vi "Timer Get Time.vi"(8 "error in (no error)":errorcluster, 11 "Timer reference":refnum<data-value>) -> (0 "error out":errorcluster, 1 "Running ?":bool, 2 "Elapsed Time (ms)":u32, 3 "Timer reference  out":refnum<data-value>)   [LabVIEW 2018]
doc: "This VI is part of a Timer class that is implemented with the DVR. It returns current values of the timer while the Timer is running.\n\nAAL 9/09"
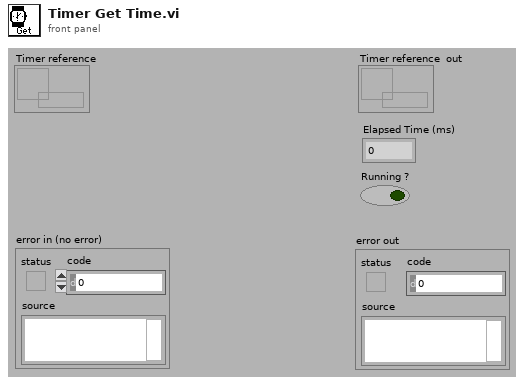
[diagram p1: front panel]
types:
  T1 = cluster{"Start Time":i32, "Elapsed Time":i32, "Running?":bool}
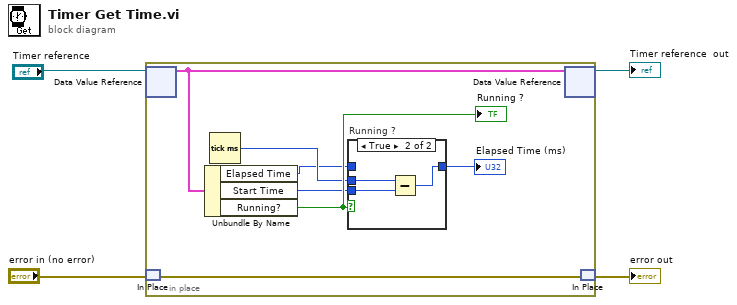
[diagram p0: block diagram]
diagram:
  n1 = in-place {
    n2 = in-place-dvr #1("Timer reference") -> (w5:T1)  [unwired: 1 out]
    n3 = in-place-match #2("error in (no error)") -> (w11:errorcluster)
    n4 = Unbundle By Name(w5) -> ("Elapsed Time"=w6:i32, "Start Time"=w7:i32, "Running?"=w9:bool)
    "Running ?" <- w9
    n5 = Tick Count (ms)() -> (millisecond timer value=w8:u32)
    n6 = case "Running ?" shown="True" w9 {
      tunnel: w8 -> [_ w15]
      tunnel: w7 -> [_ w14]
      tunnel: [w12 w13] -> w10
      tunnel: w6 -> [w12 _]
      frame False {
      }
      frame True {
        n7 = Subtract(x=w15, y=w14) -> (x-y=w13:u32)
      }
    }
    "Elapsed Time (ms)" <- w10
    n8 = in-place-dvr #1(w5) -> (→"Timer reference  out":refnum<data-value>)  [unwired: 1 out]
    n9 = in-place-match #2(w11) -> (→"error out":errorcluster)
  }
